vi "Layout - UTC frame agreement.vi"(8 "error in (no error)":errorcluster) -> (0 "error out":errorcluster)   [LabVIEW 2026, in "Tests.lvlib"]
doc: "Unit test (Caraya) for per-appender useUTC frame agreement.\nFor one appender, the file-name timestamp, the calendar-folder date, and the layout line timestamp must all render in the same time frame (UTC or local) selected by useUTC, per SRS-LMBR-036. The test uses an instant near UTC midnight so UTC and local fall on different dates on a non-UTC machine, which makes a frame mismatch observable.\nWith useUTC=TRUE the three renderings all match the known UTC date; with useUTC=FALSE they agree with each other (local frame, asserted by mutual agreement so it stays timezone-independent).\nPure test: calls FormatTimeString, ISO8601FileName, and BaseFolder directly; no actors, no file I/O.\n\nImplements LMBR-T-038 -> SRS-011, SRS-035, SRS-036. Assert-level IDs: Test-ID-Assert-Checklist.md."
uses:
  Tests.lvlib
  <vilib>/addons/_JKI Toolkits/Caraya/classes/Assert/Assert Equal Value_Variant.vi
  <vilib>/addons/_JKI Toolkits/Caraya/classes/Test/Test.lvclass
  src/Lumberjack.lvlib
  <vilib>/addons/_JKI Toolkits/Caraya/classes/Assert/Assert.lvclass
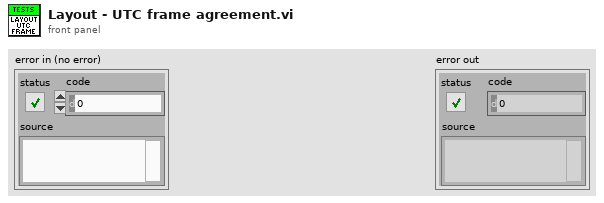
[diagram p1: front panel]
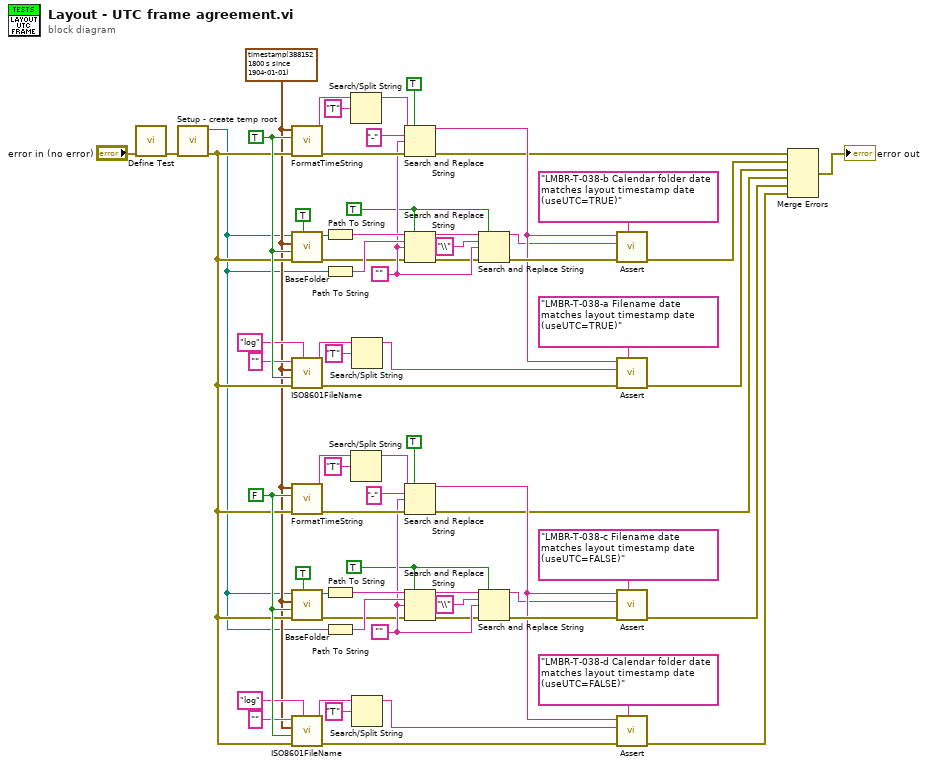
[diagram p0: block diagram]
diagram:
  w18 = TRUE ("replace all? (F)")
  w20 = ""
  w33 = FALSE ("useUTC")
  w49 = TRUE ("replace all? (F)")
  w51 = ""
  w64 = TRUE ("useUTC")
  w5 = timestamp(3881521800 s since 1904-01-01)
  n1 = call <vilib>:"Define Test.vi"("error in (no error)"="error in (no error)") -> ("error out"=w66:errorcluster)  [unwired: 9 in, 1 out]
  n2 = call "Setup - create temp root.vi"("error in (no error)"=w66) -> ("error out"=w6:errorcluster, "tempRoot"=w4:path)  [unwired: 9 in]
  n3 = call "FormatTimeString.vi"("error in (no error)"=w6, "useUTC"=w64, "timestamp"=w5) -> ("error out"=w58:errorcluster, "timeString"=w61:string)  [unwired: 7 in]
  n4 = call "BaseFolder.vi"("calendarFolderTree"=TRUE, "error in (no error)"=w6, "useUTC"=w64, "Timestamp"=w5, "RootFolder"=w4) -> ("error out"=w46:errorcluster, "Folder"=w55:path)  [unwired: 5 in]
  n5 = call "ISO8601FileName.vi"("Extension"="log", "error in (no error)"=w6, "useUTC"=w64, "Timestamp"=w5, "BaseName"="") -> ("error out"=w43:errorcluster, "FileName"=w47:string)  [unwired: 5 in]
  n6 = call "FormatTimeString.vi"("error in (no error)"=w6, "useUTC"=w33, "timestamp"=w5) -> ("error out"=w27:errorcluster, "timeString"=w30:string)  [unwired: 7 in]
  n7 = call "BaseFolder.vi"("calendarFolderTree"=TRUE, "error in (no error)"=w6, "useUTC"=w33, "Timestamp"=w5, "RootFolder"=w4) -> ("error out"=w15:errorcluster, "Folder"=w24:path)  [unwired: 5 in]
  n8 = call "ISO8601FileName.vi"("Extension"="log", "error in (no error)"=w6, "useUTC"=w33, "Timestamp"=w5, "BaseName"="") -> ("error out"=w12:errorcluster, "FileName"=w16:string)  [unwired: 5 in]
  n9 = Path To String(path=w55) -> (string=w54:string)
  n10 = Path To String(path=w4) -> (string=w53:string)
  n11 = Path To String(path=w24) -> (string=w23:string)
  n12 = Path To String(path=w4) -> (string=w22:string)
  n13 = Search/Split String(string=w61, search string/char (-)="T") -> (substring before match=w59:string)  [unwired: 1 in, 2 out]
  n14 = Search/Split String(string=w30, search string/char (-)="T") -> (substring before match=w28:string)  [unwired: 1 in, 2 out]
  n15 = Search/Split String(string=w47, search string/char (-)="T") -> (substring before match=w42:string)  [unwired: 1 in, 2 out]
  n16 = Search/Split String(string=w16, search string/char (-)="T") -> (substring before match=w11:string)  [unwired: 1 in, 2 out]
  n17 = Search and Replace String(replace all?=TRUE ("replace all? (F)"), input string=w59, search string="-" ("substring (\"\")"), replace string=w51, error in=w58) -> (result string=w41:string, error out=w39:errorcluster)  [unwired: 3 in, 2 out]
  n18 = Search and Replace String(replace all?=w49, input string=w54, search string=w53, replace string=w51, error in=w46) -> (result string=w50:string, error out=w45:errorcluster)  [unwired: 3 in, 2 out]
  n19 = Search and Replace String(replace all?=TRUE ("replace all? (F)"), input string=w28, search string="-" ("substring (\"\")"), replace string=w20, error in=w27) -> (result string=w10:string, error out=w3:errorcluster)  [unwired: 3 in, 2 out]
  n20 = Search and Replace String(replace all?=w18, input string=w23, search string=w22, replace string=w20, error in=w15) -> (result string=w19:string, error out=w14:errorcluster)  [unwired: 3 in, 2 out]
  n21 = Search and Replace String(replace all?=w49, input string=w50, search string="\\", replace string=w51, error in=w45) -> (result string=w40:string, error out=w44:errorcluster)  [unwired: 3 in, 2 out]
  n22 = Search and Replace String(replace all?=w18, input string=w19, search string="\\", replace string=w20, error in=w14) -> (result string=w9:string, error out=w13:errorcluster)  [unwired: 3 in, 2 out]
  n23 = call-poly <vilib>:"Assert.vi"("Label"="LMBR-T-038-b Calendar folder date matches layout timestamp date (useUTC=TRUE)", "error in (no error)"=w44, "Actual"=w40, "Expected"=w41) -> ("error out"=w38:errorcluster)  [unwired: 6 in, 1 out]
  n24 = call-poly <vilib>:"Assert.vi"("Label"="LMBR-T-038-a Filename date matches layout timestamp date (useUTC=TRUE)", "error in (no error)"=w43, "Actual"=w42, "Expected"=w41) -> ("error out"=w37:errorcluster)  [unwired: 6 in, 1 out]
  n25 = call-poly <vilib>:"Assert.vi"("Label"="LMBR-T-038-c Filename date matches layout timestamp date (useUTC=FALSE)", "error in (no error)"=w13, "Actual"=w9, "Expected"=w10) -> ("error out"=w2:errorcluster)  [unwired: 6 in, 1 out]
  n26 = call-poly <vilib>:"Assert.vi"("Label"="LMBR-T-038-d Calendar folder date matches layout timestamp date (useUTC=FALSE)", "error in (no error)"=w12, "Actual"=w11, "Expected"=w10) -> ("error out"=w1:errorcluster)  [unwired: 6 in, 1 out]
  n27 = Merge Errors(w39, w38, w37, w3, w2, w1) -> (→"error out":errorcluster)
